vi "Dialog - Configure Test Parameters.vi"(1 "Experiment Parameter Values (default)":T1(array[cluster])) -> (0 "Experiment Parameter Values (default) 2":T1(array[cluster]))   [LabVIEW 2011, in "Core SubVIs.lvlib"]
uses:
  Core SubVIs.lvlib
  Instance           2 42Saved   Dialog - Configure Test Parameters .vi
  Instance           1 42Saved   Dialog - Configure Test Parameters .vi
panel:
  in  "Save Parameter Value File":bool
  in  "Load Parameter Value File":bool
  in  "Color Values":u32[](array[colorbox])
  in  "Float Values":dbl[][](array[numeric]) format="%.2f"
  in  "Test Parameters Table":i32(listbox)
  in  "Cancel Button":bool
  in  "Apply Button":bool
  out "error out":errorcluster
  in  "error in (no error)":errorcluster
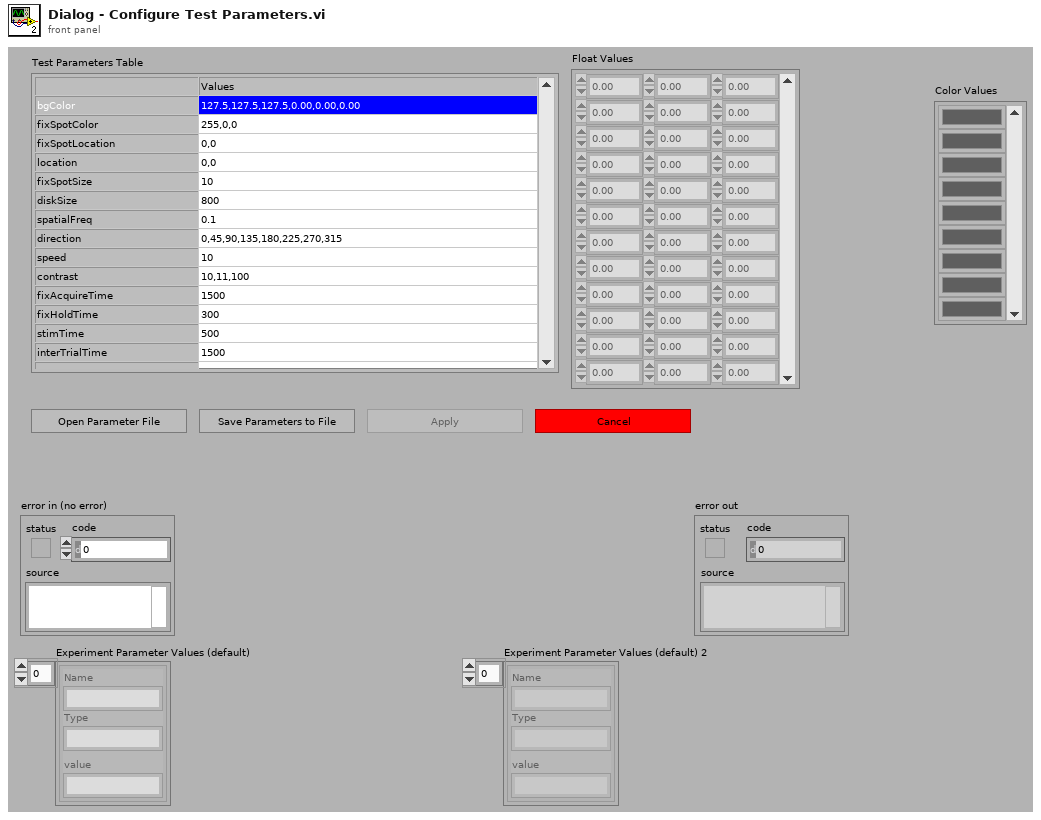
[diagram p1: front panel]
types:
  T1 = cluster{"Name":string, "Type":string, "value":string}[]
  T2 = cluster{"Name":string, "Type":string, "value":string}
  T3 = cluster{"String":string, "Type":string, "value":string}[]
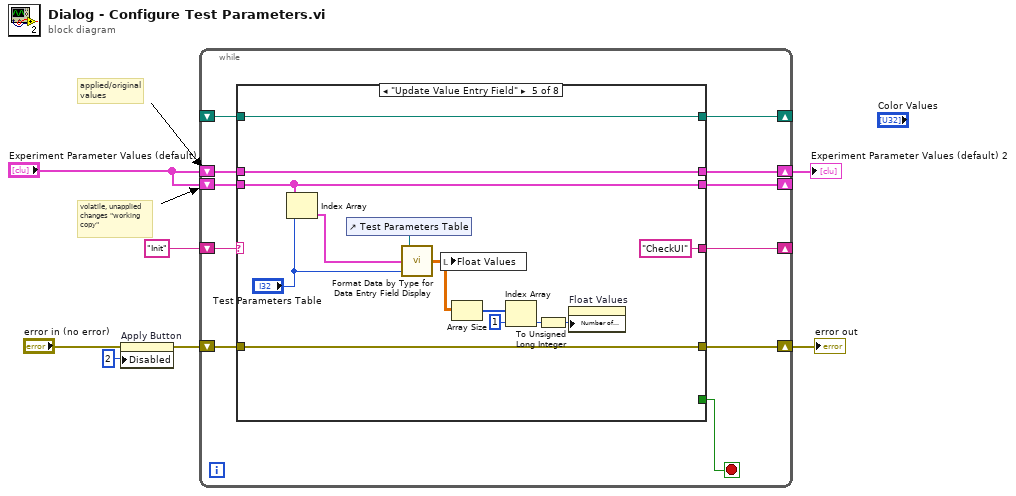
[diagram p0: block diagram]
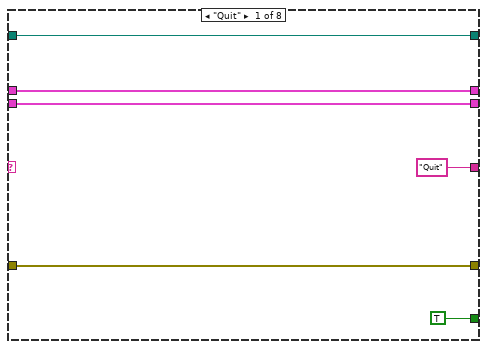
[diagram p2: hidden frame]
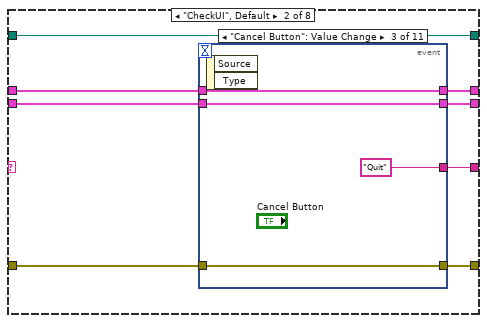
[diagram p3: hidden frame]
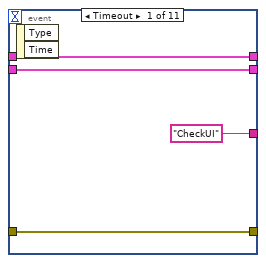
[diagram p4: hidden frame]
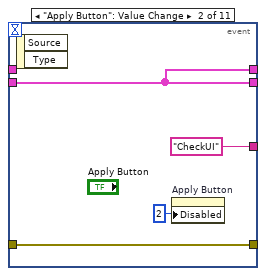
[diagram p5: hidden frame]
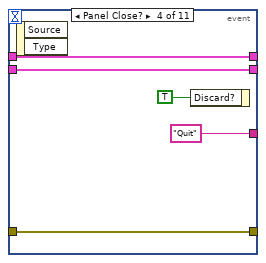
[diagram p6: hidden frame]
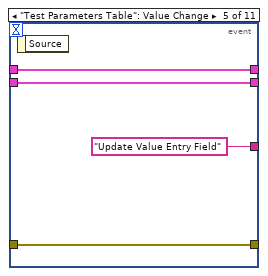
[diagram p7: hidden frame]
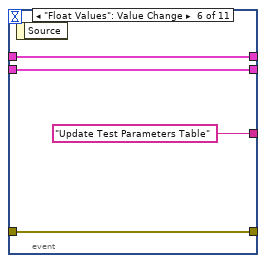
[diagram p8: hidden frame]
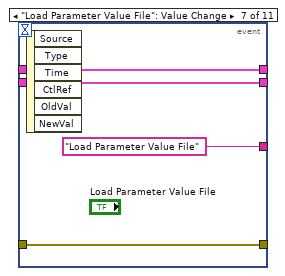
[diagram p9: hidden frame]
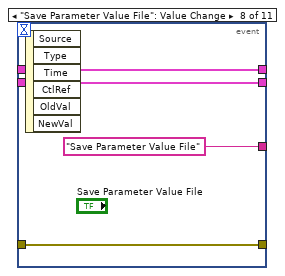
[diagram p10: hidden frame]
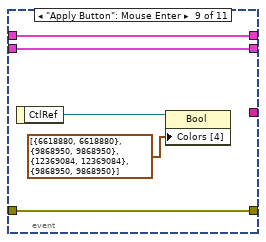
[diagram p11: hidden frame]
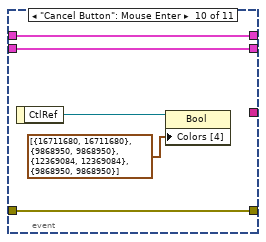
[diagram p12: hidden frame]
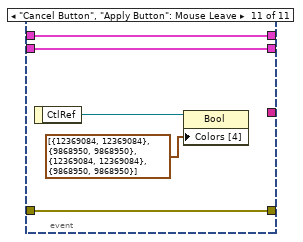
[diagram p13: hidden frame]
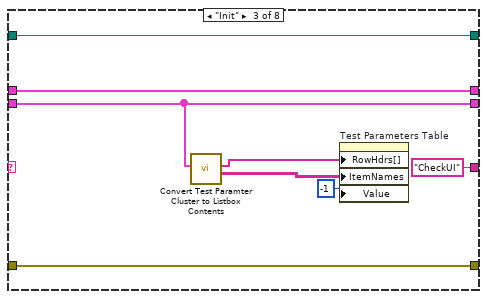
[diagram p14: hidden frame]
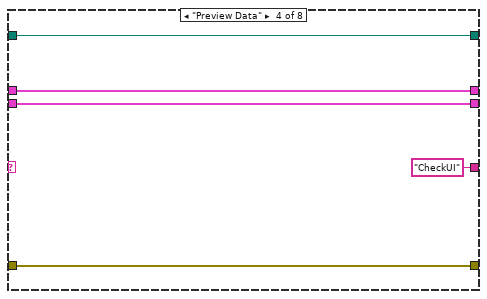
[diagram p15: hidden frame]
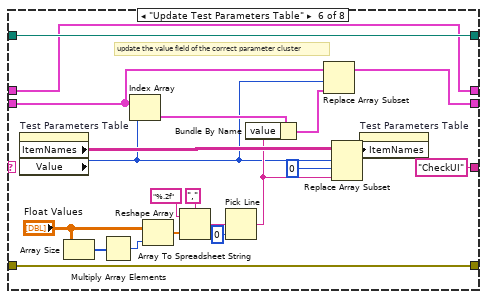
[diagram p16: hidden frame]
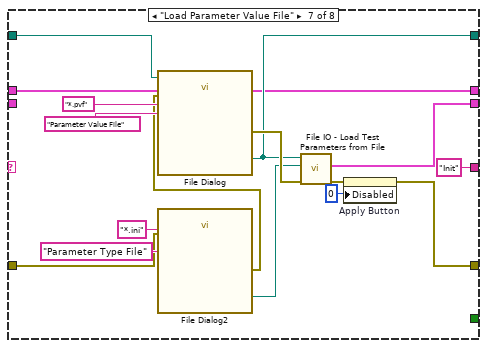
[diagram p17: hidden frame]
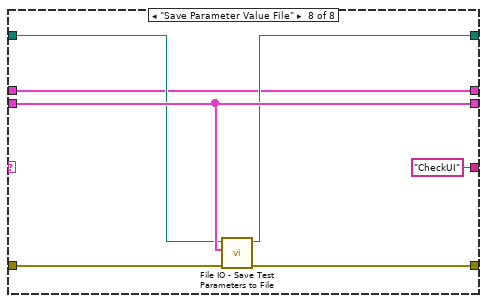
[diagram p18: hidden frame]
diagram:
  # "volatile, unapplied\nchanges \"working\ncopy\""
  # "applied/original\nvalues"
  n1 = property on="Apply Button" class="Bool"(error in="error in (no error)", "Disabled"=u8 2) -> (error out=w2:errorcluster)  [unwired: 1 in, 1 out]
  n2 = while {
    shift-right: [w17] -> _
    shift-left: "Init" -> [w18]
    shift-right: [w14] -> _
    shift-left: "Experiment Parameter Values (default)" -> [w15]
    shift-right: [w12] -> w6
    shift-left: w2 -> [w11]
    shift-right: [w10] -> _
    shift-left: _ -> [w9]
    shift-right: [w8] -> w1
    shift-left: "Experiment Parameter Values (default)" -> [w13]
    stop <- w16 stop-if-true
    n3 = case shown="\"Update Value Entry Field\"" w18 {
      tunnel: ["Quit" w30 "CheckUI" "CheckUI" "CheckUI" "CheckUI" "Init" "CheckUI"] -> w17
      tunnel: [TRUE _ _ _ _ _ _ _] -> w16
      tunnel: w15 -> [w22 w31 w85 w93 w104 w112 _ w149]
      tunnel: [w22 w32 w85 w93 w104 w109 w139 w149] -> w14
      tunnel: w13 -> [w19 w26 w81 w89 w94 w107 w128 w144]
      tunnel: [w21 w29 w87 w91 w105 w126 w129 w147] -> w12
      tunnel: w11 -> [w21 w28 w87 w91 w105 w126 w135 w148]
      tunnel: [w20 w27 w82 w90 w95 w108 w133 w145] -> w10
      tunnel: w9 -> [w20 w27 w82 w90 w95 w108 w132 w146]
      tunnel: [w19 w25 w81 w89 w94 w107 w128 w144] -> w8
      frame "Quit" {
      }
      frame "CheckUI", Default {
        n4 = event shown="[2] \"Cancel Button\": Value Change" {
          selector: _ -> [_ _ _ _ _ _ _ _ _ _ _]
          dyn-events: _ -> [_ _ _ _ _ _ _ _ _ _ _]
          timeout: _ -> [_ _ _ _ _ _ _ _ _ _ _]
          tunnel: [w36 w37 w41 w45 w51 w55 w59 w63 w70 w75 w80] -> w32
          tunnel: w31 -> [w36 w37 w41 w45 w51 w55 w59 w63 w70 w75 w80]
          tunnel: ["CheckUI" "CheckUI" "Quit" "Quit" "Update Value Entry Field" "Update Test Parameters Table" "Load Parameter Value File" "Save Parameter Value File" _ _ _] -> w30
          tunnel: w26 -> [w33 _ w42 w46 w50 w54 w58 w62 w66 w71 w76]
          tunnel: [w34 w39 w43 w47 w52 w56 w60 w64 w68 w73 w78] -> w29
          tunnel: w28 -> [w34 w39 w43 w47 w52 w56 w60 w64 w68 w73 w78]
          tunnel: [w33 w37 w42 w46 w50 w54 w58 w62 w66 w71 w76] -> w25
          event Timeout {
            n5 = event-data() -> ()  [unwired: 3 out]
          }
          event "Apply Button": Value Change {
            n6 = event-data() -> ()  [unwired: 3 out]
            n7 = property on="Apply Button" class="Bool"("Disabled"=u8 2) -> ()  [unwired: 2 in, 2 out]
          }
          event "Cancel Button": Value Change {
            n8 = event-data() -> ()  [unwired: 3 out]
          }
          event Panel Close? {
            n9 = event-data() -> ()  [unwired: 3 out]
            n10 = event-data("Discard?"=TRUE) -> ()  [unwired: 1 in, 1 out]
          }
          event "Test Parameters Table": Value Change {
            n11 = event-data() -> ()  [unwired: 2 out]
          }
          event "Float Values": Value Change {
            n12 = event-data() -> ()  [unwired: 2 out]
          }
          event "Load Parameter Value File": Value Change {
            n13 = event-data() -> ()  [unwired: 7 out]
          }
          event "Save Parameter Value File": Value Change {
            n14 = event-data() -> ()  [unwired: 7 out]
          }
          event "Apply Button": Mouse Enter {
            n15 = event-data() -> ("CtlRef"=w69:refnum<vi>)  [unwired: 1 out]
            n16 = property class="Bool"(reference=w69, "Colors [4]"=cluster{u32, u32}[] [{6618880, 6618880}, {9868950, 9868950}, {12369084, 12369084}, {9868950, 9868950}]) -> ()  [unwired: 1 in, 2 out]
          }
          event "Cancel Button": Mouse Enter {
            n17 = event-data() -> ("CtlRef"=w74:refnum<vi>)  [unwired: 1 out]
            n18 = property class="Bool"(reference=w74, "Colors [4]"=cluster{u32, u32}[] [{16711680, 16711680}, {9868950, 9868950}, {12369084, 12369084}, {9868950, 9868950}]) -> ()  [unwired: 1 in, 2 out]
          }
          event "Cancel Button", "Apply Button": Mouse Leave {
            n19 = event-data() -> ("CtlRef"=w79:refnum<vi>)  [unwired: 1 out]
            n20 = property class="Bool"(reference=w79, "Colors [4]"=cluster{u32, u32}[] [{12369084, 12369084}, {9868950, 9868950}, {12369084, 12369084}, {9868950, 9868950}]) -> ()  [unwired: 1 in, 2 out]
          }
        }
      }
      frame "Init" {
        n21 = call "Convert Test Paramter Cluster to Listbox Contents.vi"("Experiment Parameter Values (default)"=w85) -> ("2D String Array"=w84:string[][], "Parameter Names"=w83:string[])  [unwired: 1 in, 8 out]
        n22 = property on="Test Parameters Table" class="MCListbox (strict)"("RowHdrs[]"=w83, "ItemNames"=w84, "Value"=-1 ("Multicolumn Listbox")) -> ()  [unwired: 2 in, 2 out]
      }
      frame "Preview Data" {
      }
      frame "Update Value Entry Field" {
        n23 = Index Array(array=w104, index="Test Parameters Table") -> (element=w102:T2)
        n24 = control-ref of="Test Parameters Table"() -> (w101:refnum<vi>)
        n25 = call "Format Data by Type for Data Entry Field Display.vi"("Test Parameters Table"="Test Parameters Table", "Cluster"=w102, "MCListbox Refnum"=w101) -> ("array type (2D Dbl)"=w100:dbl[][])
        n26 = local write "Float Values"(w100) -> ()
        n27 = Array Size(array=w100) -> (size(s)=w99:i32[])
        n28 = Index Array(array=w99, index=1) -> (element=w97:i32)
        n29 = To Unsigned Long Integer(number=w97) -> (unsigned 32bit integer=w96:u32)
        n30 = property on="Float Values" class="Arr (strict)"("Number of Columns"=w96) -> ()  [unwired: 2 in, 2 out]
      }
      frame "Update Test Parameters Table" {
        # "update the value field of the correct parameter cluster"
        n31 = property on="Test Parameters Table" class="MCListbox (strict)"() -> ("ItemNames"=w125:string[][], "Value"=w110:i32)  [unwired: 2 in, 2 out]
        n32 = Array Size(array="Float Values") -> (size(s)=w115:i32[])
        n33 = Multiply Array Elements(1:w115) -> (0:w116:i32)
        n34 = Index Array(array=w112, index=w110) -> (element=w114:T2)
        n35 = Reshape Array("Float Values", w116) -> (w118:dbl[])
        n36 = Array To Spreadsheet String(delimiter (Tab)=",", array=w118, 3:"%.2f" ("format string")) -> (spreadsheet string=w121:string)
        n37 = Pick Line(multi-line string=w121, line index=0) -> (output string=w113:string)  [unwired: 1 out]
        n38 = Bundle By Name(cluster=w114, "value"=w113) -> (w111:T2)
        n39 = Replace Array Subset(array=w112, new element=w111, index=w110) -> (w109:T1)
        n40 = Replace Array Subset(array=w125, new element=w113, index (row)=w110, index (col)=0 ("disabled index (col)")) -> (w119:string[][])
        n41 = property on="Test Parameters Table" class="MCListbox (strict)"("ItemNames"=w119) -> ()  [unwired: 2 in, 2 out]
      }
      frame "Load Parameter Value File" {
        n42 = call "File Dialog2"("error in"=w135, "pattern (all files)"="*.ini", "pattern label"="Parameter Type File") -> ("selected path"=w136:path, "error out"=w134:errorcluster)  [unwired: 4 in, 7 out]
        n43 = call "File Dialog"("start path"=w132, "error in"=w134, "pattern (all files)"="*.pvf", "pattern label"="Parameter Value File") -> ("selected path"=w133:path, "error out"=w143:errorcluster)  [unwired: 3 in, 7 out]
        n44 = call "File IO - Load Test Parameters from File.vi"("error in (no error)"=w143, "Parameter Definition File"=w136, "Paramater Value File"=w133) -> ("error out"=w130:errorcluster, "Experiment Parameter Values"=w139:T3)  [unwired: 7 out]
        n45 = property on="Apply Button" class="Bool"(error in=w130, "Disabled"=u8 0) -> (error out=w129:errorcluster)  [unwired: 1 in, 1 out]
      }
      frame "Save Parameter Value File" {
        n46 = call "File IO - Save Test Parameters to File.vi"("error in"=w148, "Experiment Parameter Values (default)"=w149, "start path"=w146) -> ("error out"=w147:errorcluster, "selected path"=w145:path)  [unwired: 7 out]
      }
    }
  }
  "error out" <- w6
  "Experiment Parameter Values (default) 2" <- w1
